vi "(範例)Mecanum Steering.vi"() -> ()   [LabVIEW 2015]
doc: "This example demonstrates how to create a mecanum steering robot and use \"Apply Velocity to Wheels.vi\" to convert from the robot center velocity to wheel angular velocities."
uses:
  <vilib>/robotics/Steering/Wheel/Wheel Parameters.ctl
  <vilib>/robotics/Steering/Wheel/Rotation Direction.ctl
  <vilib>/robotics/Utilities/Visualization/Steering Visualization/Steering Picture/Draw Steering Frame Options.ctl
  <vilib>/robotics/Steering/Mecanum Wheel/Create Mecanum Wheel.vi
  <vilib>/robotics/Steering/Mecanum Steering Frame/Create Mecanum Steering Frame.vi
  <vilib>/robotics/Steering/Steering Frame/Apply Steering Frame Velocity to Wheels.vi
  <vilib>/robotics/Steering/Wheel/NI_Robotics_Wheel.lvclass
  <vilib>/robotics/Steering/Mecanum Wheel/NI_Robotics_Mecanum Wheel.lvclass
  <vilib>/robotics/Steering/Steering Frame/NI_Robotics_Steering Frame.lvclass
  <vilib>/robotics/Utilities/Visualization/Steering Visualization/Steering Picture/NI_Robotics_Steering Picture.lvlib
  <vilib>/robotics/Steering/Mecanum Steering Frame/NI_Robotics_Mecanum Steering Frame.lvclass
panel:
  out "Rear Right":dbl format="%#.2g"
  out "Front Right":dbl format="%#.2g"
  out "Rear Left":dbl format="%#.2g"
  out "Front Left":dbl format="%#.2g"
  out "picture":picture
  in  "stop":bool
  in  "Angular Velocity (rad/s)":dbl(slide) min=-5.0 max=5.0 scale=1.0..-1.0
  in  "Forward Velocity (m/s)":dbl(slide) min=-5.0 max=5.0 scale=-1.0..1.0
  in  "Lateral Velocity (m/s)":dbl(slide) min=-5.0 max=5.0 scale=-1.0..1.0
  # "This VI demonstrates how to convert from robot velocity to wheel velocities for a mecanum steering robot.\n\nRun the VI, then move the sliders to control the forward, lateral, and angular velocity components of the robot.  The Forward Wheel Velocity indicators show the velocities of the front left, front right, rear left, and rear right wheels."
  # "Steering Frame Velocity"
  # "Forward Wheel Velocities (rad/s)"
  # "Velocity component of the steering frame in the right direction (90 degrees cw from forward)."
  # "Velocity component of the steering frame in the forward direction."
  # "Angular velocity of the steering frame in the counterclockwise direction."
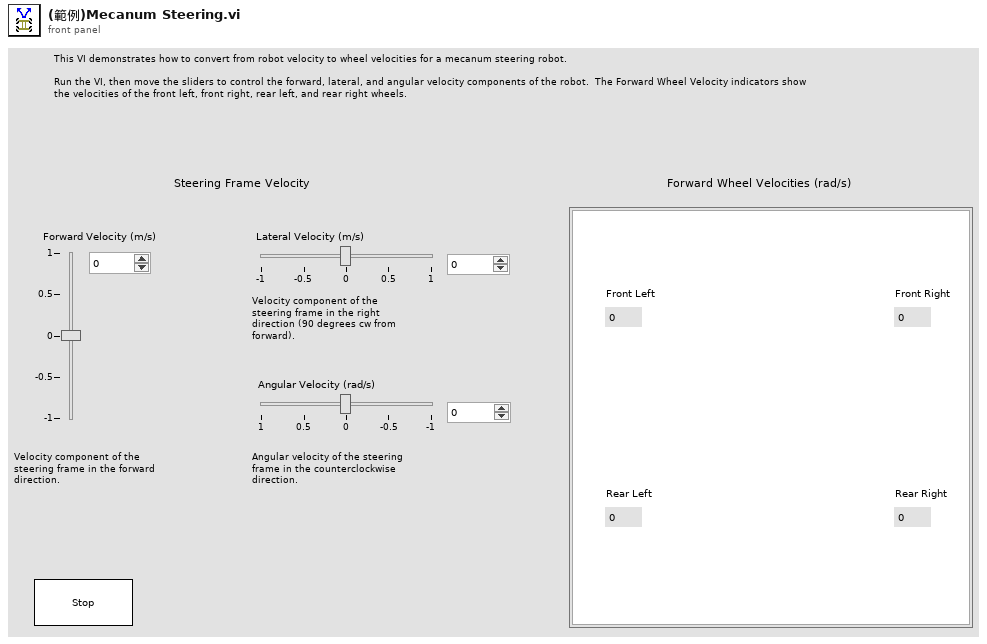
[diagram p1: front panel]
types:
  T1 = typedef "NI_Robotics_Wheel.lvclass/Wheel Parameters.ctl" = cluster{"wheel radius":dbl, "gear ratio":dbl, "forward rotation direction":T2}
  T2 = typedef "NI_Robotics_Wheel.lvclass/Rotation Direction.ctl" = u16
  T3 = cluster{"mecanum wheel out":refnum<class "NI_Robotics_Mecanum Wheel.lvclass">, "mecanum wheel out":refnum<class "NI_Robotics_Mecanum Wheel.lvclass">, "mecanum wheel out":refnum<class "NI_Robotics_Mecanum Wheel.lvclass">, "mecanum wheel out":refnum<class "NI_Robotics_Mecanum Wheel.lvclass">}
  T4 = typedef "LVBoundsTypeDef.ctl" = cluster{"Width":u32, "Height":u32}
  T5 = typedef "NI_Robotics_Steering Picture.lvlib/Draw Steering Frame Options.ctl" = cluster{"draw wheel states?":bool, "highlight wheel index":i32, "pixels per unit":dbl, "draw forward velocity?":bool, "velocity scale":dbl}
  T6 = typedef "NI_Robotics_Wheel.lvclass/Wheel State.ctl" = cluster{"wheel name":string, "forward angular velocity":dbl, "caster angular velocity":dbl, "caster wheel angle (rad)":dbl, "steering angle (rad)":dbl}
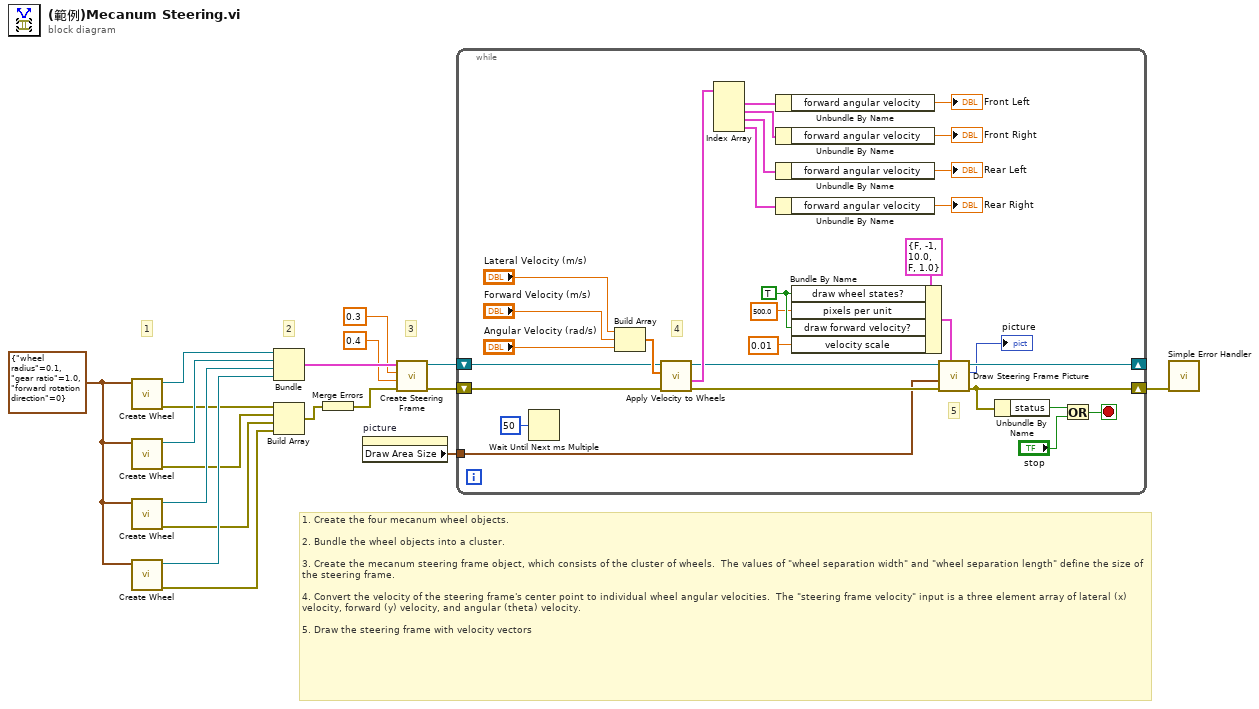
[diagram p0: block diagram]
diagram:
  w18 = T1 {"wheel radius"=0.1, "gear ratio"=1.0, "forward rotation direction"=0} ("wheel parameters")
  # "3"
  # "2"
  # "1"
  # "1. Create the four mecanum wheel objects.\n\n2. Bundle the wheel objects into a cluster.\n\n3. Create the mecanum steering frame object, which consists of the cluster of wheels.  The values of \"wheel separation width\" and \"wheel separation length\" define the size of the steering frame.\n\n4. Convert the velocity of the steering frame's center point to individual wheel angular velocities.  The \"steering frame velocity\" input is a three element array of lateral (x) velocity, forward (y) velocity, and angular (theta) velocity.\n\n5. Draw the steering frame with velocity vectors"
  n1 = call-poly <vilib>:"Create Wheel.vi"("wheel parameters"=w18) -> ("error out"=w7:errorcluster, "mecanum wheel out"=w17:refnum<class "NI_Robotics_Mecanum Wheel.lvclass">)  [unwired: 9 in]
  n2 = call-poly <vilib>:"Create Wheel.vi"("wheel parameters"=w18) -> ("error out"=w6:errorcluster, "mecanum wheel out"=w16:refnum<class "NI_Robotics_Mecanum Wheel.lvclass">)  [unwired: 9 in]
  n3 = call-poly <vilib>:"Create Wheel.vi"("wheel parameters"=w18) -> ("error out"=w5:errorcluster, "mecanum wheel out"=w15:refnum<class "NI_Robotics_Mecanum Wheel.lvclass">)  [unwired: 9 in]
  n4 = call-poly <vilib>:"Create Wheel.vi"("wheel parameters"=w18) -> ("error out"=w3:errorcluster, "mecanum wheel out"=w14:refnum<class "NI_Robotics_Mecanum Wheel.lvclass">)  [unwired: 9 in]
  n5 = Bundle("mecanum wheel out"=w17, "mecanum wheel out"=w16, "mecanum wheel out"=w15, "mecanum wheel out"=w14) -> (w13:T3)  [unwired: 1 in]
  n6 = Build Array(w7, w6, w5, w3) -> (w4:errorcluster[])
  n7 = Merge Errors(w4) -> (w2:errorcluster)
  n8 = property on="picture" class="Pict"() -> ("Draw Area Size"=w1:T4)  [unwired: 2 in, 2 out]
  n9 = call-poly <vilib>:"Create Steering Frame.vi"("error in (no error)"=w2, "wheel separation length"=0.4, "wheel separation width"=0.3, "wheels"=w13) -> ("error out"=w9:errorcluster, "mecanum steering frame out"=w10:refnum<class "NI_Robotics_Mecanum Steering Frame.lvclass">)  [unwired: 6 in]
  n10 = while {
    shift-right: [w33] -> _
    shift-left: w10 -> [w35]
    shift-right: [w32] -> w8
    shift-left: w9 -> [w34]
    tunnel: w1 -> [w28]
    stop <- w38 stop-if-true
    w21 = TRUE ("draw wheel states")
    # "5"
    # "4"
    n11 = Wait Until Next ms Multiple(millisecond multiple=u32 50) -> ()  [unwired: 1 out]
    n12 = Build Array("Lateral Velocity (m/s)", "Forward Velocity (m/s)", "Angular Velocity (rad/s)") -> (w37:dbl[])
    n13 = call-poly <vilib>:"Apply Velocity to Wheels.vi"("error in (no error)"=w34, "steering frame velocity"=w37, "steering frame in"=w35) -> ("error out"=w29:errorcluster, "calculated wheel states"=w36:T6[], "steering frame out"=w30:refnum<class "NI_Robotics_Mecanum Steering Frame.lvclass">)  [unwired: 5 in, 1 out]
    n14 = Index Array(array=w36) -> (element #1=w47:T6, element #2=w44:T6, element #3=w45:T6, element #4=w46:T6)  [unwired: 4 in]
    n15 = Unbundle By Name(w47) -> ("forward angular velocity"=→"Front Left":dbl)
    n16 = Unbundle By Name(w44) -> ("forward angular velocity"=→"Front Right":dbl)
    n17 = Unbundle By Name(w45) -> ("forward angular velocity"=→"Rear Left":dbl)
    n18 = Unbundle By Name(w46) -> ("forward angular velocity"=→"Rear Right":dbl)
    n19 = Bundle By Name(cluster=T5 {"draw wheel states?"=FALSE, "highlight wheel index"=-1, "pixels per unit"=10.0, "draw forward velocity?"=FALSE, "velocity scale"=1.0} ("draw options"), "draw wheel states?"=w21, "pixels per unit"=500.0 ("pixels per unit (10)"), "draw forward velocity?"=w21, "velocity scale"=0.01 ("velocity scale (1)")) -> (w19:T5)
    n20 = call <vilib>:"Draw Steering Frame Picture.vi"("drawing options"=w19, "error in (no error)"=w29, "picture draw area size (pixels)"=w28, "steering frame in"=w30) -> ("error out"=w32:errorcluster, "picture out"=→"picture":picture, "steering frame out"=w33:refnum<class "NI_Robotics_Mecanum Steering Frame.lvclass">)  [unwired: 5 in]
    n21 = Unbundle By Name(w32) -> ("status"=w40:bool)
    n22 = Or(x=w40, y="stop") -> (x .or. y?=w38:bool)
  }
  n23 = call <vilib>:"Simple Error Handler.vi"("error in (no error)"=w8) -> ()  [unwired: 4 in, 5 out]
